vi "Fiducial Match.vi"(8 "error in (no error)":errorcluster, 10 "input cluster":T1, 11 "Gantry In":refnum<k24>) -> (0 "error out":errorcluster, 1 "Not Found?":bool, 2 "output cluster":T1, 3 "Gantry Out":refnum<k24>)   [LabVIEW 2021, in "Component Tray.lvclass"]
uses:
  Component Tray.lvclass
  Find Component.ctl
  Controller/Camera/Machine Vision.ctl
  C:/Program Files (x86)/Aerotech/A3200/LabVIEW/2010/Bin/Aerotech.A3200.dll
  Program Files (x86)/Aerotech/A3200/LabVIEW/2010/Bin/Aerotech.A3200.dll
  Controller/Motion/A3200/A3200.lvclass
  Controller/Camera/Camera.lvclass
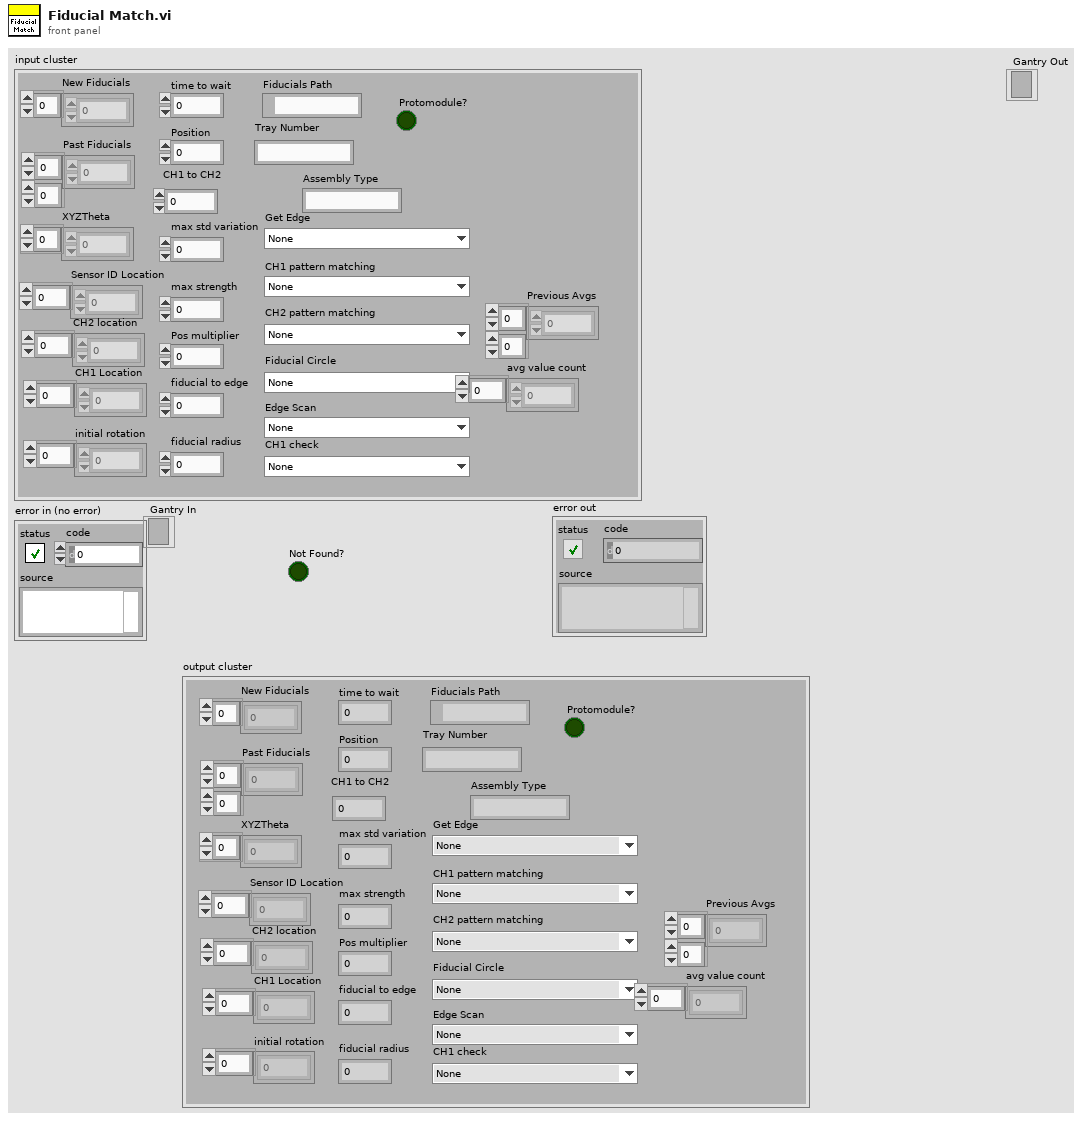
[diagram p1: front panel]
types:
  T1 = typedef "Component Tray.lvclass/Find Component.ctl" = cluster{"New Fiducials":dbl[], "Past Fiducials":dbl[][], "XYZTheta":dbl[], "Fiducials Path":path, "Position":i32, "CH1 Location":dbl[], "Sensor ID Location":dbl[], "initial rotation":dbl[], "CH2 location":dbl[], "max std variation":dbl, "max strength":dbl, "CH2 pattern matching":T2, "Fiducial Circle":T2, "Get Edge":T2, "Pos multiplier":dbl, "time to wait":u32, "fiducial to edge":dbl, "Protomodule?":bool, "Assembly Type":string, "CH1 to CH2":dbl, "Tray Number":string, "fiducial radius":dbl, "4 fiducials?":bool, "CH1 check":T2, "Edge Scan":T2, "CH1 pattern matching":T2, "Sensor Thickness":dbl, "Previous Avgs":dbl[][], "avg value count":dbl[]}
  T2 = typedef "Camera.lvclass/Machine Vision.ctl" = enum16{"None", "Assembly Tray Circle", "Assembly Tray Fiducial", "Partial Hexaboard", "sensor edge init", "HB edge init", "sensor edge pos1", "sensor edge pos2", "HB edge pos1", "HB edge pos2", "Sensor CH1-2", "HB CH1", "HB CH2", "V3 Sensor Circle", "Hexaboard Circle", "sensor CH1 check", "HB CH1 check ", "sensor ID"}
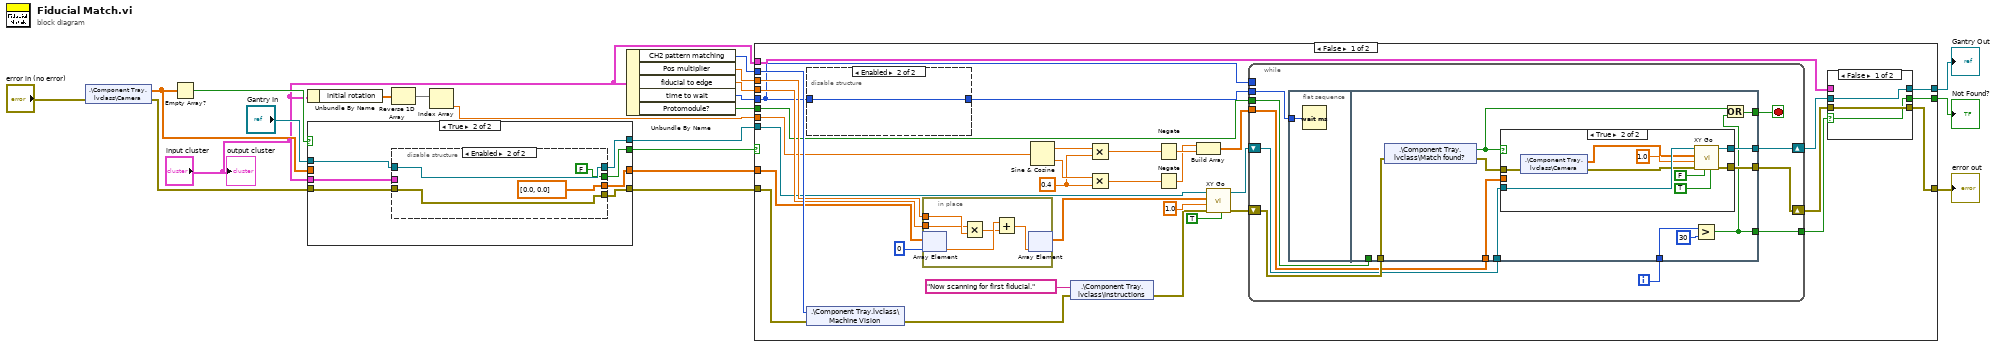
[diagram p0: block diagram]
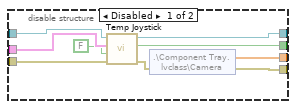
[diagram p3: hidden frame]
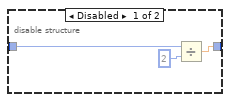
[diagram p4: hidden frame]
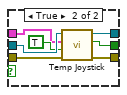
[diagram p5: hidden frame]
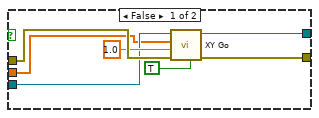
[diagram p6: hidden frame]
diagram:
  n1 = shared-variable ".\\Component Tray.lvclass\\Camera"(error in="error in (no error)") -> (w11:dbl[], error out=w7:errorcluster)
  n2 = Empty Array?(array=w11) -> (empty?=w12:bool)
  n3 = Unbundle By Name("input cluster") -> ("initial rotation"=w16:dbl[])
  n4 = case shown="True" w12 {
    selector: w12 -> [w22 _]
    tunnel: [w25 w27] -> w13
    tunnel: w11 -> [w25 _]
    tunnel: "Gantry In" -> [w24 w32]
    tunnel: [w24 w31] -> w8
    tunnel: "input cluster" -> [_ w30]
    tunnel: w7 -> [w23 w29]
    tunnel: [w23 w28] -> w6
    tunnel: [w22 w26] -> w5
    frame False {
    }
    frame True {
      n5 = disable-structure shown="Enabled" {
        disable-tunnel: w32 -> [w41 w44]
        disable-tunnel: [w40 w44] -> w31
        disable-tunnel: w30 -> [w39 _]
        disable-tunnel: w29 -> [w37 w43]
        disable-tunnel: [w35 w43] -> w28
        disable-tunnel: [w34 dbl[] [0.0, 0.0] ("Array of Double")] -> w27
        disable-tunnel: [w33 FALSE ("Error?")] -> w26
        frame Disabled {
          n6 = call "Temp Joystick.vi"("error in (no error)"=w37, "Fiducial?"=FALSE, "Component"=w39, "Gantry In"=w41) -> ("error out"=w36:errorcluster, "Error?"=w33:bool, "Gantry Out"=w40:refnum<k24>)  [unwired: 5 in]
          n7 = shared-variable ".\\Component Tray.lvclass\\Camera"(error in=w36) -> (w34:dbl[], error out=w35:errorcluster)
        }
        frame Enabled {
        }
      }
    }
  }
  n8 = Reverse 1D Array(array=w16) -> (reversed array=w17:dbl[])
  n9 = Index Array(array=w17) -> (element=w18:dbl)  [unwired: 1 in]
  n10 = Unbundle By Name("input cluster") -> ("CH2 pattern matching"=w21:T2, "Pos multiplier"=w20:dbl, "fiducial to edge"=w19:dbl, "time to wait"=w1:u32, "Protomodule?"=w10:bool)
  n11 = case shown="False" w5 {
    selector: w5 -> [_ w139]
    tunnel: w21 -> [w79 _]
    tunnel: w20 -> [w76 _]
    tunnel: w19 -> [w75 _]
    tunnel: w18 -> [w72 _]
    tunnel: [w53 w138] -> w3
    tunnel: [w52 w139] -> w15
    tunnel: w13 -> [w67 _]
    tunnel: w10 -> [w49 _]
    tunnel: [w48 w137] -> w2
    tunnel: w8 -> [w57 w138]
    tunnel: w6 -> [w56 w137]
    tunnel: "input cluster" -> [w50 _]
    tunnel: w1 -> [w46 _]
    frame False {
      w69 = 0.4 ("y")
      n12 = disable-structure shown="Enabled" {
        disable-tunnel: [w81 w83] -> w47
        disable-tunnel: w46 -> [w80 w83]
        frame Disabled {
          n13 = Divide(x=w80, y=u32 2) -> (x/y=w81:dbl)
        }
        frame Enabled {
        }
      }
      n14 = shared-variable ".\\Component Tray.lvclass\\Machine Vision"(w79, error in=w56) -> (error out=w58:errorcluster)
      n15 = in-place {
        in-place-border: w76 -> [w134]
        in-place-border: w75 -> [w133]
        n16 = in-place-array #1(w67, 0) -> (w136:dbl)
        n17 = Multiply(x=w133, y=w134) -> (x*y=w135:dbl)
        n18 = Add(x=w136, y=w135) -> (x+y=w132:dbl)
        n19 = in-place-array #1(w132) -> (w74:dbl[])  [unwired: 1 out]
      }
      n20 = Sine & Cosine(0:w72) -> (1:w71:dbl, 2:w70:dbl)
      n21 = shared-variable ".\\Component Tray.lvclass\\Instructions"("Now scanning for first fiducial." ("Instructions"), error in=w58) -> (error out=w59:errorcluster)
      n22 = Multiply(x=w71, y=w69) -> (x*y=w66:dbl)
      n23 = Multiply(x=w70, y=w69) -> (x*y=w64:dbl)
      n24 = Negate(x=w66) -> (-x=w65:dbl)
      n25 = Negate(x=w64) -> (-x=w63:dbl)
      n26 = Build Array(w63, w65) -> (w68:dbl[])
      n27 = call "XY Go.vi"("Increment?"=TRUE, "error in (no error)"=w59, "Speed"=1.0, "XY In"=w74, "Gantry In"=w57) -> ("error out"=w61:errorcluster, "Gantry Out"=w62:refnum<k24>)  [unwired: 4 in, 1 out]
      n28 = while {
        shift-right: [w99] -> w54
        shift-left: w62 -> [w102]
        shift-right: [w100] -> w51
        shift-left: w61 -> [w103]
        tunnel: w68 -> [w101]
        tunnel: [w98] -> w55
        tunnel: w49 -> [w96]
        tunnel: w47 -> [w94]
        tunnel: w46 -> [_]
        i -> [w95]
        stop <- w97 stop-if-true
        n29 = flat-sequence {
          tunnel: w94 -> [w104]
          tunnel: w103 -> [w111]
          tunnel: w102 -> [w115]
          tunnel: w101 -> [w114]
          tunnel: [w113] -> w100
          tunnel: [w112] -> w99
          tunnel: [w106] -> w98
          tunnel: [w109] -> w97
          tunnel: w96 -> [_]
          tunnel: w95 -> [w107]
          frame #0 {
            n30 = Wait (ms)(milliseconds to wait=w104) -> ()  [unwired: 1 out]
          }
          frame #1 {
            n31 = shared-variable ".\\Component Tray.lvclass\\Match found?"(error in=w111) -> (w108:bool, error out=w110:errorcluster)
            n32 = case shown="True" w108 {
              tunnel: w110 -> [w121 w131]
              tunnel: w115 -> [w119 w130]
              tunnel: [w118 w128] -> w113
              tunnel: [w117 w129] -> w112
              tunnel: w114 -> [w116 _]
              frame False {
                n33 = call "XY Go.vi"("Increment?"=TRUE, "error in (no error)"=w121, "Speed"=1.0, "XY In"=w116, "Gantry In"=w119) -> ("error out"=w118:errorcluster, "Gantry Out"=w117:refnum<k24>)  [unwired: 4 in, 1 out]
              }
              frame True {
                n34 = shared-variable ".\\Component Tray.lvclass\\Camera"(error in=w131) -> (w126:dbl[], error out=w123:errorcluster)
                n35 = call "XY Go.vi"("Increment?"=TRUE, "return immediately"=FALSE, "error in (no error)"=w123, "Speed"=1.0, "XY In"=w126, "Gantry In"=w130) -> ("error out"=w128:errorcluster, "Gantry Out"=w129:refnum<k24>)  [unwired: 3 in, 1 out]
              }
            }
            n36 = Greater?(x=w107, y=30) -> (0:w106:bool)
            n37 = Or(x=w108, y=w106) -> (x .or. y?=w109:bool)
          }
        }
      }
      n38 = case shown="False" w55 {
        selector: w55 -> [w84 _]
        tunnel: w54 -> [w86 w93]
        tunnel: [w86 w92] -> w53
        tunnel: [w84 w91] -> w52
        tunnel: w51 -> [w85 w89]
        tunnel: [w85 w88] -> w48
        tunnel: w50 -> [_ w87]
        frame False {
        }
        frame True {
          n39 = call "Temp Joystick.vi"("error in (no error)"=w89, "Fiducial?"=TRUE, "Component"=w87, "Gantry In"=w93) -> ("error out"=w88:errorcluster, "Error?"=w91:bool, "Gantry Out"=w92:refnum<k24>)  [unwired: 5 in]
        }
      }
    }
    frame True {
    }
  }
  "Gantry Out" <- w3
  "error out" <- w2
  "Not Found?" <- w15
  "output cluster" <- "input cluster"
